vi "Initial Values-Unbundler-Bool.vi"(8 "error in (no error)":errorcluster, 9 "Keys Array":T2, 10 "Section name":string, 11 "User profile ini file ref":T1) -> (0 "error out":errorcluster, 3 "User profile ini file ref":T1)   [LabVIEW 2013]
uses:
  Typedefs/Ini file interface (Boolean).ctl
  <vilib>/Utility/config.llb/Config Data RefNum.ctl
  Typedefs/HW config states enum.ctl
  Typedefs/Read Write Enum.ctl
  Global Variables/General Globals.vi
  Global Variables/gl_UI Ctrl Refs.vi
  <vilib>/Utility/config.llb/NI_LVConfig.lvlib
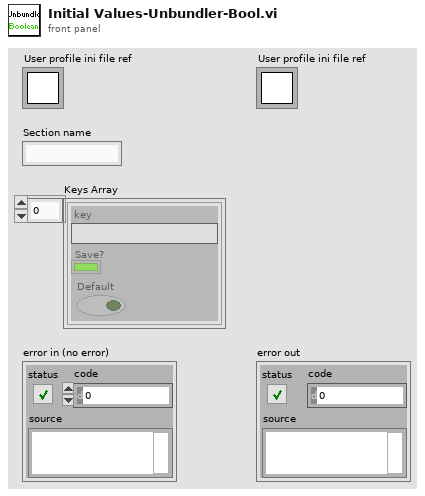
[diagram p1: front panel]
types:
  T1 = typedef "NI_LVConfig.lvlib/Config Data RefNum.ctl" = refnum<k1>
  T2 = typedef "Ini file interface (Boolean).ctl" = cluster{"key":string, "Save?":bool, "Default":bool}[]
  T3 = typedef "Read Write Enum.ctl" = enum16{"Read", "Write"}
  T4 = typedef "HW config states enum.ctl" = enum16{"Load from file", "Save to file", "Write all", "Read all", "Write XY stage settings", "Write DAQ FPGA settings", "Write Control FPGA settings", "Write Phys Channels", "Clear", "Compare from file"}
  T5 = typedef "Sys Configuration.ctl" = cluster{"XY Stage":T6, "DAQ FPGA":T7, "Control system":T11, "Encoder":T12, "DAQmx Chan":T13, "Computer MAC address":string, "Cam VidRec":T14, "Externalise Triggers":bool, "Laser wavelength (nm)":dbl}
  T6 = typedef "XY Stage config cluster.ctl" = cluster{"COM port":refnum<visa-resource-name>, "XY stage available":bool}
  T7 = typedef "DAQ FPGA config cluster.ctl" = cluster{"Ref":T8, "Target":T9, "Clock Freq (MHz) ":dbl, "input card type":T10, "Samples Wait after Trigger":u16, "AOD fill":u16, "StartupDelay":i32, "Slip Cycle (clock cycles)":u32, "Add Cycle":bool}
  T8 = typedef "FPGA Ref.ctl" = refnum<k20>
  T9 = typedef "nirio_resource_hc.ctl" = tag
  T10 = typedef "FPGA input type AC-DC.ctl" = enum16{"AC Card", "DC Card"}
  T11 = typedef "CTRL system config cluster.ctl" = cluster{"Ethernet opened":bool, "Ethernet Port":u32, "Ctrl FPGA available":bool, "Ctrl FPGA Clock (MHz)":dbl, "Ctrl system MAC address":string, "Control system.Network adapter name":string, "AOD 1 Amplitude":i16, "AOD 2 Amplitude":i16, "AOD 3 Amplitude":i16, "AOD 4 Amplitude":i16, "Data Time Interval (ns)":dbl, "T0 (ns)":dbl, "Ta (ns)":dbl}
  T12 = typedef "Encoder config cluster.ctl" = cluster{"IP address":string, "Port":u16, "Encoder available":bool, "Wheel radius (cm)":dbl}
  T13 = typedef "DAQmx physical channels cluster.ctl" = cluster{"Pockels AO":tag, "Hard shutter AO":tag, "PMT AOs":tag, "Power meter AI":tag}
  T14 = typedef "Cam VidRec HW config setup cluster.ctl" = cluster{"DO flag-Video record":tag, "DO flag-Trial start":tag, "VidRec available":bool}
  T15 = typedef "UI ctrl refs cluster.ctl" = cluster{"Top level VI path":path, "Top level VI ref":refnum<vi>, "User menu ref":refnum<k9>, "Sub Panel control":refnum<vi>, "Imaging Param Tab":refnum<vi>, "Occurrence-Start drivers":refnum<k4>, "Occurrence-Speed logging initialised":refnum<k4>, "Occurrence-XYZ stage initialised":refnum<k4>, "Exit button":refnum<vi>, "Status ind":refnum<vi>, "Return to Origin":refnum<vi>, "Speed Logging":refnum<vi>, "Time Lapse":refnum<vi>, "Live Imaging":refnum<vi>, "AOL Z Stack":refnum<vi>, "Motor Z Stack":refnum<vi>, "Funct Acq button":refnum<vi>, "Hard Shutter":refnum<vi>, "Virtual Shutter":refnum<vi>, "Laser Power":refnum<vi>, "AOL Mode":refnum<vi>, "Frame Size":refnum<vi>, "Field of View":refnum<vi>, "Dwell Time":refnum<vi>, "Zoom":refnum<vi>, "AOL Z":refnum<vi>, "Objective":refnum<vi>, "Axis":refnum<vi>, "Paths & Names":refnum<vi>, "Experiment folder path (ind.)":refnum<vi>, "Last State (Ind.)":refnum<vi>, "Laser wavelength ind (nm)":refnum<vi>, "Averages":refnum<vi>, "Angle (degrees)":refnum<vi>, "X centre":refnum<vi>, "Y centre":refnum<vi>, "Plane Mode":refnum<vi>, "# Planes":refnum<vi>, "Z Start":refnum<vi>, "Z Stop":refnum<vi>, "Z Step":refnum<vi>, "PMT 1":refnum<vi>, "PMT 2":refnum<vi>, "Stage XYZ Position":refnum<vi>, "Pockels@Z Start":refnum<vi>, "Pockels@Z Stop":refnum<vi>, "Obtain Z Start":refnum<vi>, "Obtain Z Stop":refnum<vi>, "Live stim.trig.period":refnum<vi>, "Live stim.trig.enable":refnum<vi>, "Funct. Acq. Pockels Modulation":refnum<vi>, "Enable Video Recording":refnum<vi>, "Video Record-Live Imaging":refnum<vi>, "Video Record-Funct acq":refnum<vi>, "AOL Z-stack Chirps Ready (ind)":refnum<vi>, "Center freq ind (nm)":refnum<vi>, "Logging queue (ind)":refnum<vi>, "Back aperture power (ind.)":refnum<vi>, "Power after objective (ind.)":refnum<vi>, "Switch user":refnum<vi>}
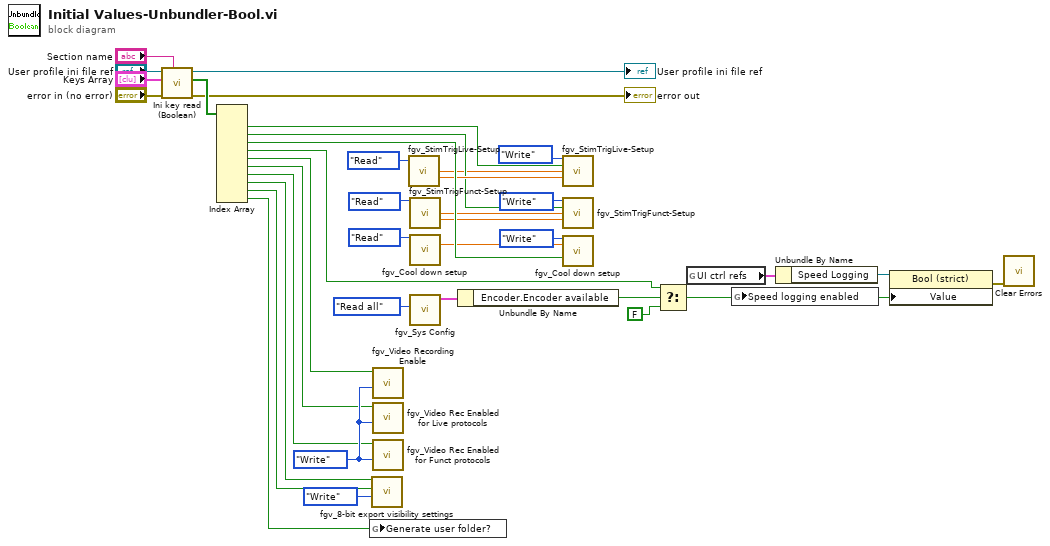
[diagram p0: block diagram]
diagram:
  w10 = Read_Write_Enum."Write" ("Function")
  n1 = call "Ini key read (Boolean).vi"("Section"="Section name", "error in (no error)"="error in (no error)", "Parameter names & setup"="Keys Array", "Ini file refnum in"="User profile ini file ref") -> ("error out"=→"error out":errorcluster, "Value read/used"=w24:bool[], "Ini file refnum out"=→"User profile ini file ref":T1)  [unwired: 5 in]
  n2 = Index Array(array=w24) -> (element #1=w28:bool, element #2=w32:bool, element #3=w38:bool, element #4=w12:bool, element #5=w6:bool, element #6=w5:bool, element #7=w4:bool, element #8=w3:bool, element #9=w2:bool, element #10=w1:bool)  [unwired: 10 in]
  n3 = global write "General Globals.vi" "Generate user folder?"(w1) -> ()
  n4 = call "fgv_8-bit export visibility settings.vi"("Function"=enum16{"Intialize", "Write", "Read", "Clear"}."Write", "Include camera videos"=w2, "Include speed graph"=w3) -> ()  [unwired: 6 in, 3 out]
  n5 = call "fgv_Video Recording Enable.vi"("Function"=w10, "Video Recording Enabled"=w6) -> ()  [unwired: 9 in, 1 out]
  n6 = call "fgv_Video Rec Enabled for Live protocols.vi"("Function"=w10, "Video Recording Enabled for Live protocols"=w5) -> ()  [unwired: 9 in, 1 out]
  n7 = call "fgv_Video Rec Enabled for Funct protocols.vi"("Function"=w10, "Video Recording Enabled for functional acq protocols"=w4) -> ()  [unwired: 9 in, 1 out]
  n8 = call "fgv_StimTrigLive-Setup.vi"("Function"=enum16{"Intialize", "Write", "Read", "Clear"}."Read") -> ("Live stim.trig.period (sec)"=w27:dbl, "Live stim.trig.width (ms)"=w33:dbl)  [unwired: 11 in, 2 out]
  n9 = call "fgv_StimTrigFunct-Setup.vi"("Function"=enum16{"Intialize", "Write", "Read", "Clear"}."Read") -> ("Funct stim.trig.delay (sec)"=w34:dbl, "Funct stim.trig.width (ms)"=w31:dbl)  [unwired: 11 in, 2 out]
  n10 = call "fgv_Cool down setup.vi"("Function"=enum16{"Intialize", "Write", "Read", "Clear"}."Read") -> ("Cool-down time (s)"=w37:dbl)  [unwired: 12 in, 2 out]
  n11 = call "fgv_Sys Config.vi"("Function"=HW_config_states_enum."Read all") -> ("System Config out"=w17:T5)  [unwired: 9 in, 1 out]
  n12 = Unbundle By Name(w17) -> ("Encoder.Encoder available"=w13:bool)
  n13 = call "fgv_StimTrigLive-Setup.vi"("Function"=enum16{"Intialize", "Write", "Read", "Clear"}."Write", "Live stim.trig.enable"=w28, "Live stim.trig.period (sec)"=w27, "Live stim.trig.width (ms)"=w33) -> ()  [unwired: 8 in, 4 out]
  n14 = call "fgv_StimTrigFunct-Setup.vi"("Function"=enum16{"Intialize", "Write", "Read", "Clear"}."Write", "Live stim.trig.enable"=w32, "Funct stim.trig.delay (sec)"=w34, "Funct stim.trig.width (ms)"=w31) -> ()  [unwired: 8 in, 4 out]
  n15 = call "fgv_Cool down setup.vi"("Function"=enum16{"Intialize", "Write", "Read", "Clear"}."Write", "Cool-down time (s)"=w37, "Enable cool-down time"=w38) -> ()  [unwired: 10 in, 3 out]
  n16 = Select(t=w12, s=w13, f=FALSE) -> (s? t:f=w8:bool)
  n17 = global read "gl_UI Ctrl Refs.vi" "UI ctrl refs"() -> (w14:T15)
  n18 = global write "General Globals.vi" "Speed logging enabled"(w8) -> ()
  n19 = Unbundle By Name(w14) -> ("Speed Logging"=w15:refnum<vi>)
  n20 = property class="Bool (strict)"(reference=w15, "Value"=w8) -> (error out=w7:errorcluster)  [unwired: 1 in, 1 out]
  n21 = call <vilib>:"Clear Errors.vi"("error in (no error)"=w7) -> ()  [unwired: 6 in, 1 out]
